vi "RIOWaveformDataStore.vi"(3 "Error in":errorcluster, 4 "Experiment State":T1={"error"={"status"=FALSE, "code"=0, "source"=""}, "Digitizer DAQmx Tasks"={"TaskArray"=[]}, "DAQ Settings"={"Channel Settings"=[], "Card Settings"=[]}, "Synchronization Settings"={"Synchronizer 0"="", "source terminal"="", "Synchronizer 1"=""}, "DAQ Data"=[], "Next Shot#"="", "System Message"="", "User Shot Notes"="", "Timing Settings"={"Timing Card Settings"=[], "Timing Channel Settings"=[]}, "Timing Tasks"={"TaskArray"=[]}, "Tree"="", "Time Card/Channels"=[], "DAQ Card/Channels"=[], "Program Version"="", "RIO Settings"={"Channel Settings"=[], "Card Settings"=[]}, "RIO References"={"Reference Array"=[]}, "RIO Data"={"RIO Deleaved Data"=[], "Raw Readout"=[]}, "RIO Card/Channels"=[], "DIO Channels"=0, "DIO Settings"={"DIO Channel Array"=[]}, "Global Settings"={"Initial Background Values"={"Reference Shot #"=0.0, "Background pressure [Torr]"=0.0, "Cryo temp [V]"=0.0, "Cryo temp [K]"=0.0, "Cryotemp Calibration File"=path ""}, "Gas Puffing"={"Gas A type"="N", "Gas B type"="N", "Gas C type"="N", "Gas A pressure [psi]"=0.0, "Gas B pressure [psi]"=0.0, "Gas C pressure [psi]"=0.0, "Innner Electrode"="", "Middle Electrode"="", "Outer Electrode"="", "Gas A bottle pressure [psi]"=0.0, "Gas B bottle pressure [psi]"=0.0, "Gas C bottle pressure [psi]"=0.0}, "PSU Voltages"={"Bias1 Voltage [V]"=0.0, "Bias2 Voltage [V]"=0.0, "PSU1 Voltage [V]"=0.0, "Puff-PSU1 CH1 Voltage [V]"=0.0, "Puff-PSU1 CH2 Voltage [V]"=0.0, "Puff-PSU1 CH3 Voltage [V]"=0.0, "PSU2 Voltage [V]"=0.0, "PSU3 Voltage [V]"=0.0}, "TEK 2024B Details"={"CH1"="", "CH2"="", "CH3"="", "CH4"="", "CH1 Ground State"="Grounded", "CH2 Ground State"="Grounded", "CH3 Ground State"="Grounded", "CH4 Ground State"="Grounded"}}, "Calibrations"={"CryoTemp"={"Comment"="", "X"=[], "Y"=[]}, "PSU2 Tach"={"Comment"="", "X"=[], "Y"=[]}, "PSU3 Tach"={"Comment"="", "X"=[], "Y"=[]}, "PSU2 RevTach"={"Comment"="", "X"=[], "Y"=[]}, "PSU3 RevTach"={"Comment"="", "X"=[], "Y"=[]}}, "Tach Tasks"={"PSU2 task"="", "PSU3 task"=""}, "PSU2 Panel Settings"={"PSU2 DIO channels"={"Charge relay DIO"="DAQ0/port0/line3", "Dump relay DIO"="DAQ0/port0/line4", "HV Arm DIO"="DAQ0/port0/line5", "HV On DIO"="DAQ0/port0/line6"}, "PSU2 Tachometer Controls"={"PSU2 Tach Calibration"=path "Z:/Data/Calibration/Tachometer", "PSU2 Charging Voltage [kV]"=0.0, "PSU2 Tach Counter"="DAQ0/port0/line3"}, "PSU2 Reverse Tachometer Controls"={"PSU2 RevTach Calibration"=path "Z:/Data/Calibration/Reverse Tachometer/PSU2_RevTachCalibration.csv", "PSU2 bank Voltage [kV]"=0.0, "PSU2 RevTach Counter"=""}}, "PSU3 Panel Settings"={"PSU3 DIO channels"={"Charge relay DIO"="DAQ0/port0/line5", "Dump relay DIO"="DAQ0/port0/line6", "HV Arm DIO"="", "HV On DIO"="DAQ0/port0/line6"}, "PSU3 Tachometer Controls"={"PSU3 Tach Calibration"=path "Z:/Data/Calibration/Reverse Tachometer/PSU3_RevTachCalibration.csv", "PSU3 Charging Voltage [kV]"=0.0, "PSU3 Tach Counter"=""}, "PSU3 Reverse Tachometer Controls"={"PSU3 RevTach Calibration"=path "Z:/Data/Calibration/Reverse Tachometer/PSU3_RevTachCalibration.csv", "PSU3 bank Voltage [kV]"=0.0, "PSU3 RevTach Counter"=""}}} {"Global Settings"."Initial Background Values"."Cryo temp [K]" format="%#_4g"; "RIO Settings"."Card Settings"."Sample Rate" format="%#_3p"; "Timing Settings"."Timing Channel Settings"."FrontPanelTime" format="%.3p"; "Timing Settings"."Timing Channel Settings"."Pulse width (s)" format="%.3p"; "Timing Settings"."Timing Channel Settings"."Delay (s)" format="%.3p"; "DAQ Settings"."Card Settings"."Global Edge Type" items=["Rising"=10280, "Falling"=10171]; "DAQ Settings"."Card Settings"."Sample Rate" format="%#_3p"}, 5 "Tree DVR in":refnum<data-value>) -> (0 "Error out":errorcluster)   [LabVIEW 2015]
uses:
  <vilib>/MDSplus/Classes/Tree_Class/Tree.lvclass
  Controls/ExperimentStateCluster.ctl
  Controls/DigitizerSettingsChannelSettings.ctl
  Controls/DigitizerSettingsCardSettingsArray.ctl
  Controls/DigitizerSettingsCardSettings.ctl
  Controls/TimingSettings.ctl
  Controls/TimingCardSettings.ctl
  Controls/TimingChannelSettings.ctl
  Controls/RIOSettingsExperimentStateCluster.ctl
  Controls/RIOChannelSettingsArrayExperimentStateCluster.ctl
  Controls/RIOSettingsChannelSettings.ctl
  Controls/RIOSettingsCardSettingsArray.ctl
  Controls/RIOSettingsCardSettings.ctl
  <vilib>/userdefined/High Color/nirio_resource_hc.ctl
  Controls/RIOData.ctl
  Controls/DIOChannel.ctl
  Controls/Global Settings/GlobalSettings.ctl
  Controls/Global Settings/InitialBackgroundValues.ctl
  Controls/Global Settings/GasPuffing.ctl
  Controls/Global Settings/PSUVoltages.ctl
  Controls/Global Settings/ScopeDetails.ctl
  Controls/Calibrations/Calibrations.ctl
  Controls/Calibrations/CryoTemoCalibration.ctl
  Controls/Calibrations/PSU2TachCalibration.ctl
  Controls/Calibrations/PSU3TachCalibration.ctl
  Controls/TachTasks.ctl
  Controls/PSU2PanelSettings.ctl
  Controls/PSU2DIOChannels.ctl
  Controls/PSU2TachometerControls.ctl
  Controls/PSU2ReverseTachometerControls.ctl
  Controls/PSU3PanelSettings.ctl
  Controls/PSU3DIOChannels.ctl
  Controls/PSU3TachometerControls.ctl
  Controls/PSU3ReverseTachometerControls.ctl
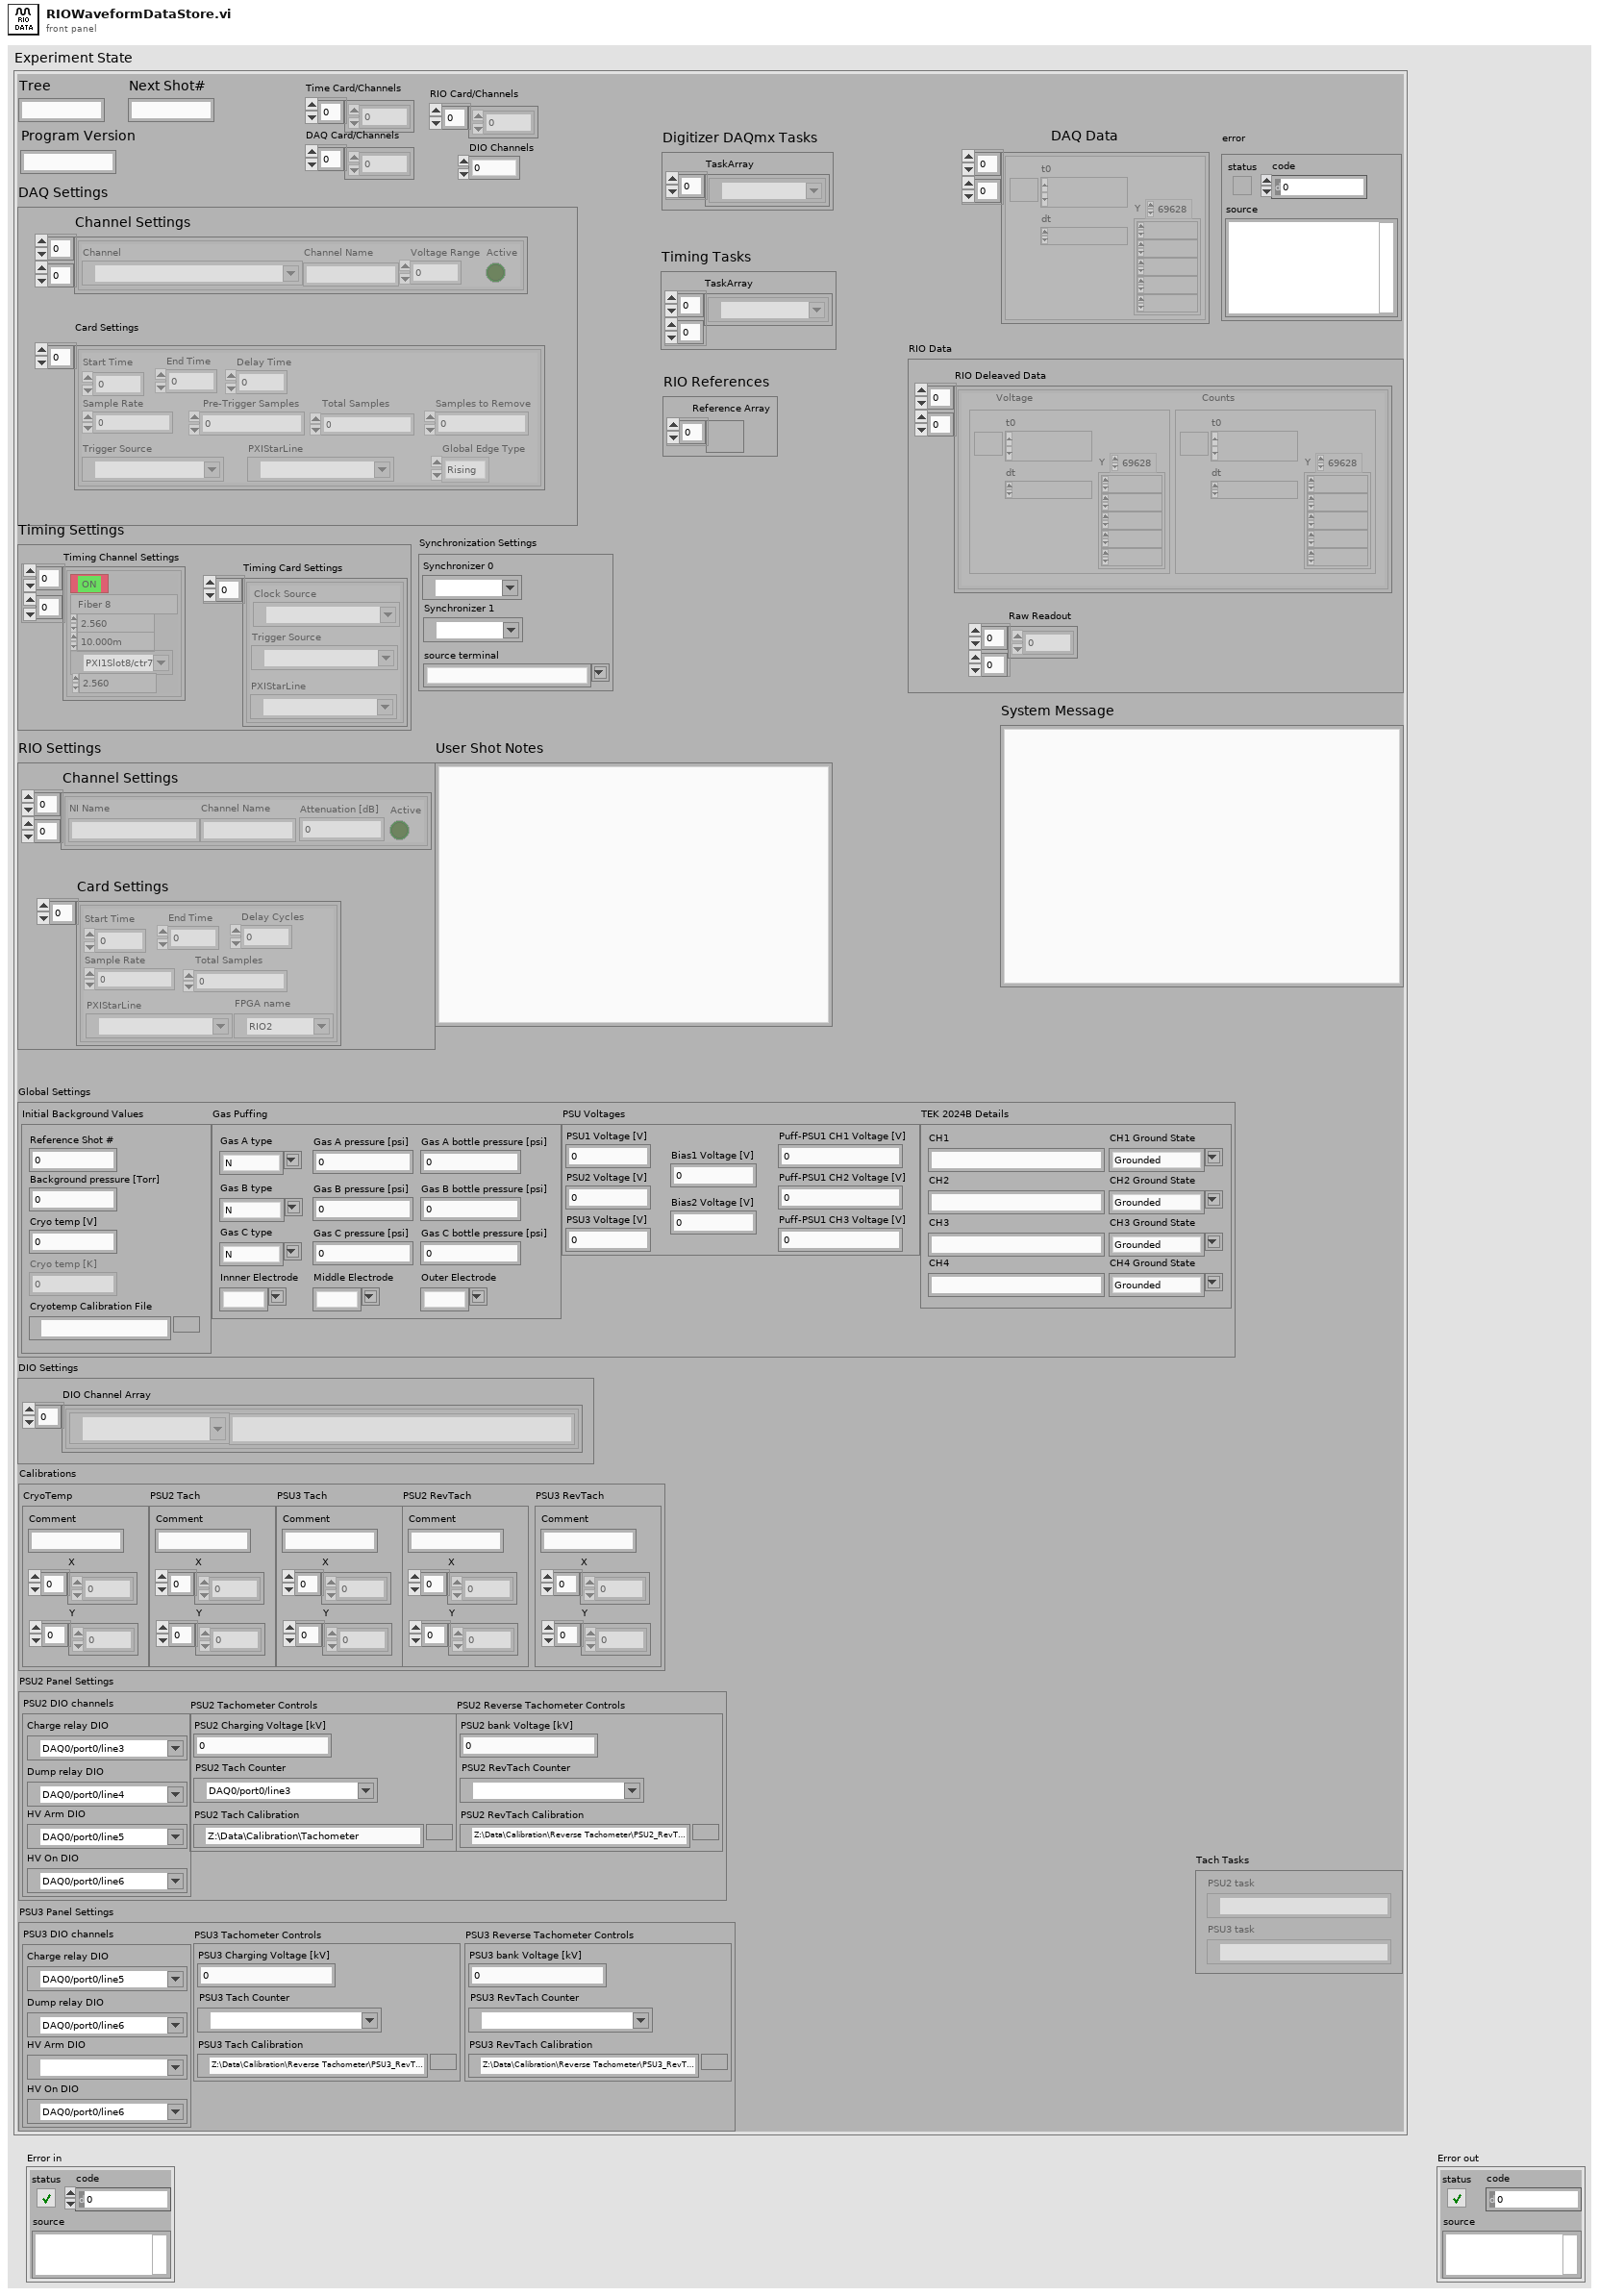
[diagram p1: front panel]
types:
  T1 = typedef "ExperimentStateCluster.ctl" = cluster{"error":errorcluster, "Digitizer DAQmx Tasks":cluster{"TaskArray":refnum<k21>[]}, "DAQ Settings":cluster{"Channel Settings":T2[][], "Card Settings":T3}, "Synchronization Settings":cluster{"Synchronizer 0":refnum<k15>, "source terminal":string, "Synchronizer 1":refnum<k15>}, "DAQ Data":waveform(dbl)[][], "Next Shot#":string, "System Message":string, "User Shot Notes":string, "Timing Settings":T5, "Timing Tasks":cluster{"TaskArray":refnum<k21>[][]}, "Tree":string, "Time Card/Channels":i32[], "DAQ Card/Channels":i32[], "Program Version":string, "RIO Settings":T8, "RIO References":cluster{"Reference Array":refnum<k20>[]}, "RIO Data":T14, "RIO Card/Channels":i32[], "DIO Channels":i32, "DIO Settings":cluster{"DIO Channel Array":T15[]}, "Global Settings":T16, "Calibrations":T21, "Tach Tasks":T25, "PSU2 Panel Settings":T26, "PSU3 Panel Settings":T30}
  T2 = typedef "DigitizerSettingsChannelSettings.ctl" = cluster{"Channel":tag, "Channel Name":string, "Voltage Range":dbl, "Active":bool}
  T3 = typedef "DigitizerSettingsCardSettingsArray.ctl" = T4[]
  T4 = typedef "DigitizerSettingsCardSettings.ctl" = cluster{"Start Time":dbl, "End Time":dbl, "Sample Rate":dbl, " Pre-Trigger Samples":u32, "Total Samples":i32, "Samples to Remove":u32, "Trigger Source":tag, "Global Edge Type":i32, "PXIStarLine":tag, "Delay Time":dbl}
  T5 = typedef "TimingSettings.ctl" = cluster{"Timing Card Settings":T6[], "Timing Channel Settings":T7[][]}
  T6 = typedef "TimingCardSettings.ctl" = cluster{"Trigger Source":tag, "Clock Source":tag, "PXIStarLine":tag}
  T7 = typedef "TimingChannelSettings.ctl" = cluster{"Delay (s)":dbl, "Pulse width (s)":dbl, "Active":bool, "Channel Name":string, "counter":tag, "FrontPanelTime":dbl}
  T8 = typedef "RIOSettingsExperimentStateCluster.ctl" = cluster{"Channel Settings":T9, "Card Settings":T11}
  T9 = typedef "RIOChannelSettingsArrayExperimentStateCluster.ctl" = T10[][]
  T10 = typedef "RIOSettingsChannelSettings.ctl" = cluster{"Channel Name":string, "Active":bool, "NI Name":string, "Attenuation [dB]":i32}
  T11 = typedef "RIOSettingsCardSettingsArray.ctl" = T12[]
  T12 = typedef "RIOSettingsCardSettings.ctl" = cluster{"Start Time":dbl, "End Time":dbl, "Sample Rate":dbl, "Total Samples":u64, "PXIStarLine":tag, "Delay Cycles":u64, "FPGA name":T13}
  T13 = typedef "nirio_resource_hc.ctl" = tag
  T14 = typedef "RIOData.ctl" = cluster{"RIO Deleaved Data":cluster{"Voltage":waveform(dbl), "Counts":waveform(i16)}[][], "Raw Readout":u64[][]}
  T15 = typedef "DIOChannel.ctl" = cluster{"Channel Name":string, "NI Name":tag}
  T16 = typedef "GlobalSettings.ctl" = cluster{"Initial Background Values":T17, "Gas Puffing":T18, "PSU Voltages":T19, "TEK 2024B Details":T20}
  T17 = typedef "InitialBackgroundValues.ctl" = cluster{"Reference Shot #":dbl, "Background pressure [Torr]":dbl, "Cryo temp [V]":dbl, "Cryo temp [K]":dbl, "Cryotemp Calibration File":path}
  T18 = typedef "GasPuffing.ctl" = cluster{"Gas A type":string, "Gas B type":string, "Gas C type":string, "Gas A pressure [psi]":dbl, "Gas B pressure [psi]":dbl, "Gas C pressure [psi]":dbl, "Innner Electrode":string, "Middle Electrode":string, "Outer Electrode":string, "Gas A bottle pressure [psi]":dbl, "Gas B bottle pressure [psi]":dbl, "Gas C bottle pressure [psi]":dbl}
  T19 = typedef "PSUVoltages.ctl" = cluster{"Bias1 Voltage [V]":dbl, "Bias2 Voltage [V]":dbl, "PSU1 Voltage [V]":dbl, "Puff-PSU1 CH1 Voltage [V]":dbl, "Puff-PSU1 CH2 Voltage [V]":dbl, "Puff-PSU1 CH3 Voltage [V]":dbl, "PSU2 Voltage [V]":dbl, "PSU3 Voltage [V]":dbl}
  T20 = typedef "ScopeDetails.ctl" = cluster{"CH1":string, "CH2":string, "CH3":string, "CH4":string, "CH1 Ground State":string, "CH2 Ground State":string, "CH3 Ground State":string, "CH4 Ground State":string}
  T21 = typedef "Calibrations.ctl" = cluster{"CryoTemp":T22, "PSU2 Tach":T23, "PSU3 Tach":T24, "PSU2 RevTach":T23, "PSU3 RevTach":T24}
  T22 = typedef "CryoTemoCalibration.ctl" = cluster{"Comment":string, "X":dbl[], "Y":dbl[]}
  T23 = typedef "PSU2TachCalibration.ctl" = cluster{"Comment":string, "X":dbl[], "Y":dbl[]}
  T24 = typedef "PSU3TachCalibration.ctl" = cluster{"Comment":string, "X":dbl[], "Y":dbl[]}
  T25 = typedef "TachTasks.ctl" = cluster{"PSU2 task":refnum<k21>, "PSU3 task":refnum<k21>}
  T26 = typedef "PSU2PanelSettings.ctl" = cluster{"PSU2 DIO channels":T27, "PSU2 Tachometer Controls":T28, "PSU2 Reverse Tachometer Controls":T29}
  T27 = typedef "PSU2DIOChannels.ctl" = cluster{"Charge relay DIO":tag, "Dump relay DIO":tag, "HV Arm DIO":tag, "HV On DIO":tag}
  T28 = typedef "PSU2TachometerControls.ctl" = cluster{"PSU2 Tach Calibration":path, "PSU2 Charging Voltage [kV]":dbl, "PSU2 Tach Counter":tag}
  T29 = typedef "PSU2ReverseTachometerControls.ctl" = cluster{"PSU2 RevTach Calibration":path, "PSU2 bank Voltage [kV]":dbl, "PSU2 RevTach Counter":tag}
  T30 = typedef "PSU3PanelSettings.ctl" = cluster{"PSU3 DIO channels":T31, "PSU3 Tachometer Controls":T32, "PSU3 Reverse Tachometer Controls":T33}
  T31 = typedef "PSU3DIOChannels.ctl" = cluster{"Charge relay DIO":tag, "Dump relay DIO":tag, "HV Arm DIO":tag, "HV On DIO":tag}
  T32 = typedef "PSU3TachometerControls.ctl" = cluster{"PSU3 Tach Calibration":path, "PSU3 Charging Voltage [kV]":dbl, "PSU3 Tach Counter":tag}
  T33 = typedef "PSU3ReverseTachometerControls.ctl" = cluster{"PSU3 RevTach Calibration":path, "PSU3 bank Voltage [kV]":dbl, "PSU3 RevTach Counter":tag}
  T34 = cluster{"Voltage":waveform(dbl), "Counts":waveform(i16)}[][]
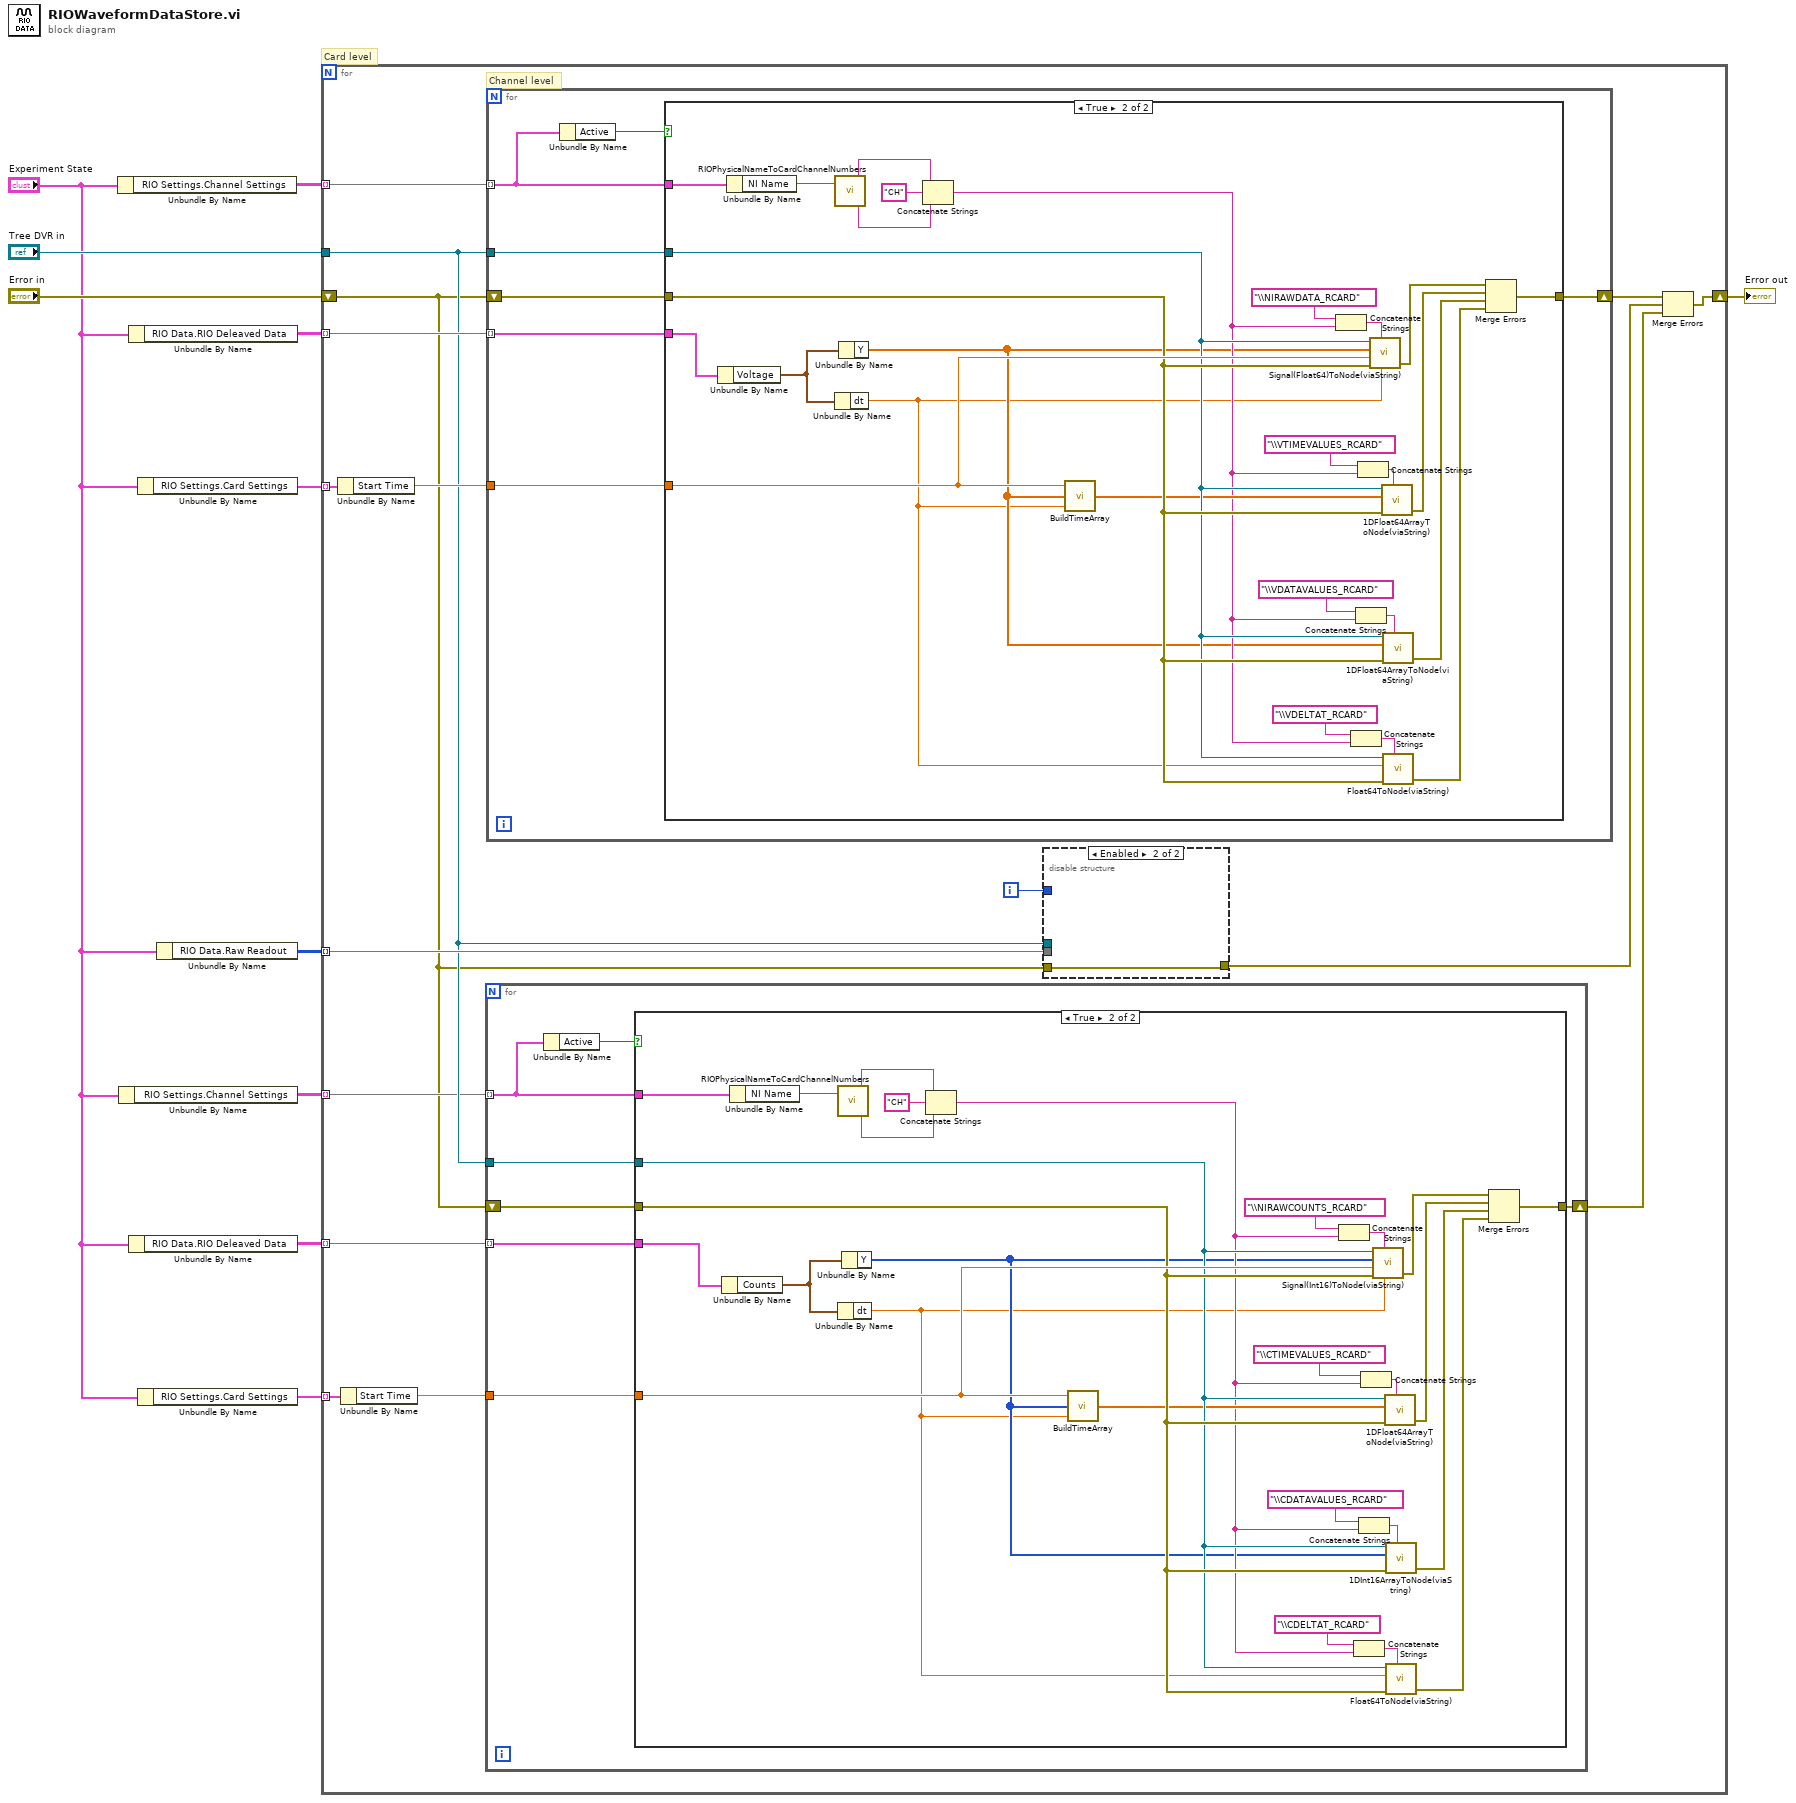
[diagram p0: block diagram]
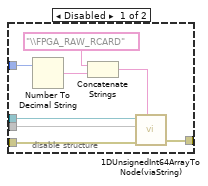
[diagram p2: hidden frame]
diagram:
  # "Card level"
  n1 = Unbundle By Name("Experiment State") -> ("RIO Settings.Channel Settings"=w7:T9)
  n2 = Unbundle By Name("Experiment State") -> ("RIO Settings.Channel Settings"=w4:T9)
  n3 = Unbundle By Name("Experiment State") -> ("RIO Data.RIO Deleaved Data"=w8:T34)
  n4 = Unbundle By Name("Experiment State") -> ("RIO Data.RIO Deleaved Data"=w3:T34)
  n5 = Unbundle By Name("Experiment State") -> ("RIO Settings.Card Settings"=w6:T11)
  n6 = Unbundle By Name("Experiment State") -> ("RIO Settings.Card Settings"=w1:T11)
  n7 = Unbundle By Name("Experiment State") -> ("RIO Data.Raw Readout"=w5:u64[][])
  n8 = for {
    tunnel: w8 -> [w27] mode=indexing
    shift-right: [w21] -> w10
    shift-left: "Error in" -> [w12]
    tunnel: "Tree DVR in" -> [w17]
    tunnel: w7 -> [w24] mode=indexing
    tunnel: w6 -> [w26] mode=indexing
    tunnel: w5 -> [w19] mode=indexing
    tunnel: w4 -> [w16] mode=indexing
    tunnel: w3 -> [w15] mode=indexing
    tunnel: w1 -> [w14] mode=indexing
    i -> [w23]
    # "Channel level"
    n9 = Unbundle By Name(w26) -> ("Start Time"=w25:dbl)
    n10 = Unbundle By Name(w14) -> ("Start Time"=w18:dbl)
    n11 = for {
      tunnel: w18 -> [w43]
      tunnel: w17 -> [w42]
      tunnel: w16 -> [w38] mode=indexing
      tunnel: w15 -> [w41] mode=indexing
      shift-right: [w40] -> w13
      shift-left: w12 -> [w39]
      n12 = Unbundle By Name(w38) -> ("Active"=w37:bool)
      n13 = case shown="True" w37 {
        tunnel: w41 -> [_ w71]
        tunnel: w39 -> [w44 w68]
        tunnel: w43 -> [_ w70]
        tunnel: w38 -> [_ w69]
        tunnel: w42 -> [_ w67]
        tunnel: [w44 w66] -> w40
        frame False {
        }
        frame True {
          n14 = Unbundle By Name(w71) -> ("Counts"=w65:waveform(i16))
          n15 = Unbundle By Name(w69) -> ("NI Name"=w61:string)
          n16 = call "RIOPhysicalNameToCardChannelNumbers.vi"("Channel Name"=w61) -> ("Channel #"=w58:string, "Card #"=w59:string)  [unwired: 1 in]
          n17 = Unbundle By Name(w65) -> ("dt"=w45:dbl)
          n18 = Unbundle By Name(w65) -> ("Y"=w47:i16[])
          n19 = Concatenate Strings(w59, "CH" ("string"), w58) -> (w48:string)
          n20 = call "BuildTimeArray.vi"("Time Increment (dt)"=w45, "Data Array (y-values)"=w47, "Start Time (t_o)"=w70) -> ("Time Array (x-values)"=w62:dbl[])
          n21 = Concatenate Strings("\\NIRAWCOUNTS_RCARD" ("string"), w48) -> (w57:string)
          n22 = Concatenate Strings("\\CDELTAT_RCARD" ("string"), w48) -> (w53:string)
          n23 = Concatenate Strings("\\CDATAVALUES_RCARD" ("string"), w48) -> (w54:string)
          n24 = Concatenate Strings("\\CTIMEVALUES_RCARD" ("string"), w48) -> (w64:string)
          n25 = call "Signal(Int16)ToNode(viaString).vi"("Tree DVR in"=w67, "NodePath"=w57, "y-axis (Data Range)"=w47, "Start Time"=w70, "Delta t"=w45, "Error in"=w68) -> ("Error out"=w56:errorcluster)  [unwired: 2 in]
          n26 = call "1DFloat64ArrayToNode(viaString).vi"("Tree DVR in"=w67, "DBL Array"=w62, "error in (no error)"=w68, "NodePath"=w64) -> ("error out"=w55:errorcluster)  [unwired: 3 in]
          n27 = call "1DInt16ArrayToNode(viaString).vi"("Tree DVR in"=w67, "I16 array in"=w47, "error in (no error)"=w68, "NodePath"=w54) -> ("error out"=w51:errorcluster)  [unwired: 3 in]
          n28 = call "Float64ToNode(viaString).vi"("Tree DVR in"=w67, "DBL in"=w45, "error in"=w68, "NodePath"=w53) -> ("error out"=w50:errorcluster)  [unwired: 3 in]
          n29 = Merge Errors(w56, w55, w51, w50) -> (w66:errorcluster)
        }
      }
    }
    n30 = for {
      tunnel: w27 -> [w78] mode=indexing
      tunnel: w25 -> [w77]
      tunnel: w24 -> [w73] mode=indexing
      tunnel: w17 -> [w75]
      shift-right: [w76] -> w22
      shift-left: w12 -> [w74]
      n31 = Unbundle By Name(w73) -> ("Active"=w72:bool)
      n32 = case shown="True" w72 {
        tunnel: w78 -> [_ w106]
        tunnel: w74 -> [w79 w103]
        tunnel: w77 -> [_ w105]
        tunnel: w73 -> [_ w104]
        tunnel: w75 -> [_ w102]
        tunnel: [w79 w101] -> w76
        frame False {
        }
        frame True {
          n33 = Unbundle By Name(w106) -> ("Voltage"=w100:waveform(dbl))
          n34 = Unbundle By Name(w104) -> ("NI Name"=w96:string)
          n35 = call "RIOPhysicalNameToCardChannelNumbers.vi"("Channel Name"=w96) -> ("Channel #"=w93:string, "Card #"=w94:string)  [unwired: 1 in]
          n36 = Unbundle By Name(w100) -> ("dt"=w80:dbl)
          n37 = Unbundle By Name(w100) -> ("Y"=w82:dbl[])
          n38 = Concatenate Strings(w94, "CH" ("string"), w93) -> (w83:string)
          n39 = call "BuildTimeArray.vi"("Time Increment (dt)"=w80, "Data Array (y-values)"=w82, "Start Time (t_o)"=w105) -> ("Time Array (x-values)"=w97:dbl[])
          n40 = Concatenate Strings("\\NIRAWDATA_RCARD" ("string"), w83) -> (w92:string)
          n41 = Concatenate Strings("\\VDELTAT_RCARD" ("string"), w83) -> (w88:string)
          n42 = Concatenate Strings("\\VDATAVALUES_RCARD" ("string"), w83) -> (w89:string)
          n43 = Concatenate Strings("\\VTIMEVALUES_RCARD" ("string"), w83) -> (w99:string)
          n44 = call "Signal(Float64)ToNode(viaString).vi"("Tree DVR in"=w102, "NodePath"=w92, "y-axis (Data Range)"=w82, "Start Time"=w105, "Delta t"=w80, "Error in"=w103) -> ("Error out"=w91:errorcluster)  [unwired: 2 in]
          n45 = call "1DFloat64ArrayToNode(viaString).vi"("Tree DVR in"=w102, "DBL Array"=w97, "error in (no error)"=w103, "NodePath"=w99) -> ("error out"=w90:errorcluster)  [unwired: 3 in]
          n46 = call "1DFloat64ArrayToNode(viaString).vi"("Tree DVR in"=w102, "DBL Array"=w82, "error in (no error)"=w103, "NodePath"=w89) -> ("error out"=w86:errorcluster)  [unwired: 3 in]
          n47 = call "Float64ToNode(viaString).vi"("Tree DVR in"=w102, "DBL in"=w80, "error in"=w103, "NodePath"=w88) -> ("error out"=w85:errorcluster)  [unwired: 3 in]
          n48 = Merge Errors(w91, w90, w86, w85) -> (w101:errorcluster)
        }
      }
    }
    n49 = disable-structure shown="Enabled" {
      disable-tunnel: w23 -> [w35 _]
      disable-tunnel: [w31 w36] -> w20
      disable-tunnel: w19 -> [w30 _]
      disable-tunnel: w17 -> [w29 _]
      disable-tunnel: w12 -> [w28 w36]
      frame Disabled {
        n50 = Number To Decimal String(number=w35) -> (decimal integer string=w33:string)  [unwired: 1 in]
        n51 = Concatenate Strings("\\FPGA_RAW_RCARD", w33) -> (w32:string)
        n52 = call "1DUnsignedInt64ArrayToNode(viaString).vi"("Tree DVR in"=w29, "U64 array in"=w30, "error in (no error)"=w28, "NodePath"=w32) -> ("error out"=w31:errorcluster)  [unwired: 3 in]
      }
      frame Enabled {
      }
    }
    n53 = Merge Errors(w22, w20, w13) -> (w21:errorcluster)
  }
  "Error out" <- w10
